vi "Read Flow Rate.vi"(8 "error in (no error)":errorcluster, 11 "Mass Flow Controller in":refnum<class "Mass Flow Controller.lvclass">) -> (0 "error out":errorcluster, 2 "Flow Rate":dbl, 3 "Mass Flow Controller out":refnum<class "Mass Flow Controller.lvclass">)   [LabVIEW 2011, in "Mass Flow Controller.lvclass"]
uses:
  Mass Flow Controller.lvclass
  Mass Flow Controller.lvclass/Mass Flow Controller.ctl
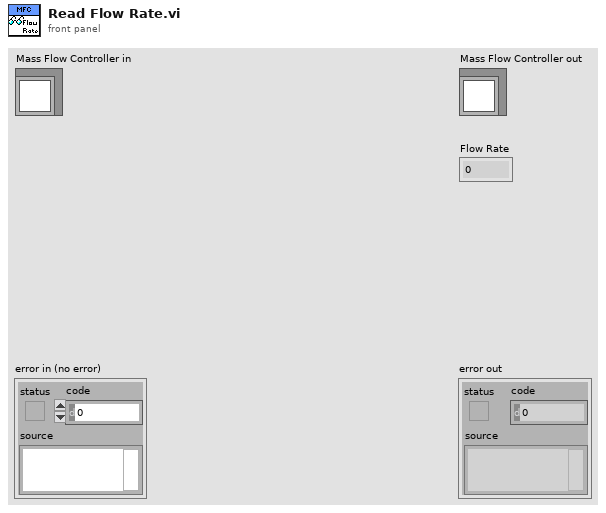
[diagram p1: front panel]
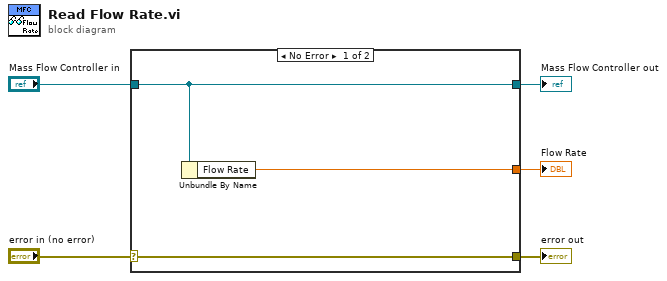
[diagram p0: block diagram]
diagram:
  n1 = case shown="No Error" "error in (no error)" {
    selector: "error in (no error)" -> [w8 w9]
    tunnel: [w8 w9] -> w4
    tunnel: [w7 w10] -> w2
    tunnel: "Mass Flow Controller in" -> [w7 w10]
    tunnel: [w6 _] -> w1
    frame No Error {
      n2 = Unbundle By Name(w7) -> ("Flow Rate"=w6:dbl)
    }
    frame Error {
    }
  }
  "error out" <- w4
  "Mass Flow Controller out" <- w2
  "Flow Rate" <- w1
